vi "Aircraft 7 Attitude Values .vi"(7 "Method":enum16{"Get", "Set"}(ring), 11 "Aircraft Att Data":T1) -> (3 "Aircraft Att Data Out":T1)   [LabVIEW 2014]
uses:
  Controls/Aircraft Attitude Data.ctl
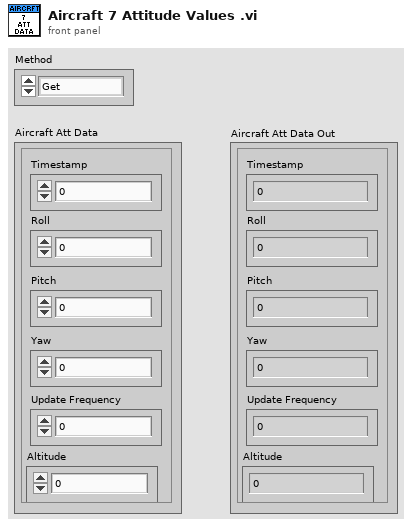
[diagram p1: front panel]
types:
  T1 = typedef "Aircraft Attitude Data.ctl" = cluster{"Roll":sgl, "Pitch":sgl, "Yaw":sgl, "Timestamp":u32, "Update Frequency":dbl, "Altitude":sgl}
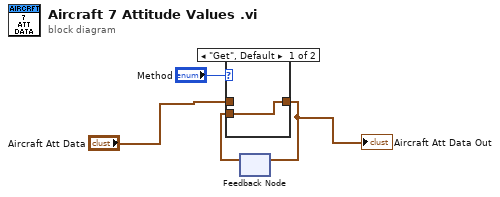
[diagram p0: block diagram]
diagram:
  n1 = feedback #1() -> (w3:T1)  [unwired: 1 in]
  n2 = case shown="\"Get\", Default" "Method" {
    tunnel: "Aircraft Att Data" -> [_ w6]
    tunnel: [w5 w6] -> w2
    tunnel: w3 -> [w5 _]
    frame "Get", Default {
    }
    frame "Set" {
    }
  }
  "Aircraft Att Data Out" <- w2
  n3 = feedback-in #1(w2) -> ()
